vi "wait.vi"(1 "State to wait for":i32, 2 "Waiting Loop ID":i32, 3 "time (ms)":i32, 4 "Current Loop ID":i32) -> (0 "Done?":bool)   [LabVIEW 2013]
doc: "This VI allows you to wait for a specified amount of time before advancing, or for a different subsystem to reach a different state. Useful in autonomous applications."
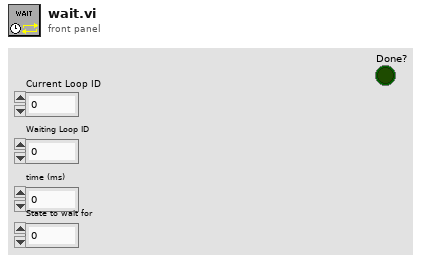
[diagram p1: front panel]
types:
  T1 = typedef "subStates.ctl" = enum16{"null", "wait", "driver control", "auto", "manual override", "hold position", "rotate", "pickup", "pass", "recover pass", "load", "goto shoot", "shoot high goal", "shoot low goal", "cancel arm", "cancel shooter", "end", "test"}
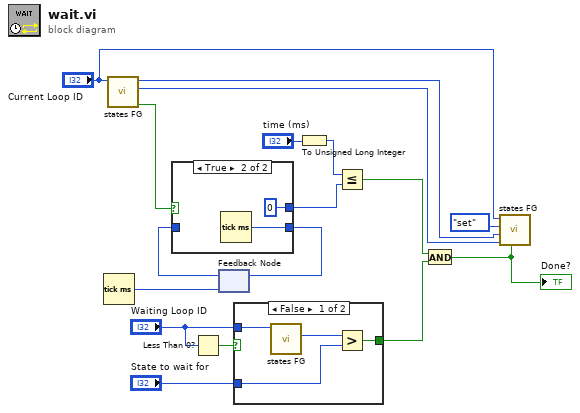
[diagram p0: block diagram]
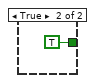
[diagram p2: hidden frame]
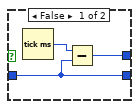
[diagram p3: hidden frame]
diagram:
  n1 = Tick Count (ms)() -> (millisecond timer value=w1:u32)
  n2 = call "states FG.vi"("Loop ID"="Current Loop ID") -> ("first call?"=w17:bool, "state # out"=w6:i32, "subState out"=w7:T1)  [unwired: 7 in, 1 out]
  n3 = Less Than 0?(x="Waiting Loop ID") -> (x < 0?=w2:bool)
  n4 = feedback #1(w1) -> (w15:u32)
  n5 = case shown="True" w17 {
    tunnel: [w19 w22] -> w16
    tunnel: w15 -> [w19 _]
    tunnel: [w18 u32 0] -> w14
    frame False {
      n6 = Tick Count (ms)() -> (millisecond timer value=w20:u32)
      n7 = Subtract(x=w20, y=w19) -> (x-y=w18:u32)
    }
    frame True {
      n8 = Tick Count (ms)() -> (millisecond timer value=w22:u32)
    }
  }
  n9 = feedback-in #1(w16) -> ()
  n10 = case shown="False" w2 {
    tunnel: "Waiting Loop ID" -> [w26 _]
    tunnel: "State to wait for" -> [w25 _]
    tunnel: [w24 TRUE] -> w11
    frame False {
      n11 = call "states FG.vi"("Loop ID"=w26) -> ("state # out"=w23:i32)  [unwired: 7 in, 3 out]
      n12 = Greater?(x=w23, y=w25) -> (0:w24:bool)
    }
    frame True {
    }
  }
  n13 = To Unsigned Long Integer(number="time (ms)") -> (unsigned 32bit integer=w4:u32)
  n14 = Less Or Equal?(x=w4, y=w14) -> (x <= y?=w12:bool)
  n15 = And(x=w12, y=w11) -> (x .and. y?=w10:bool)
  "Done?" <- w10
  n16 = call "states FG.vi"("exit in"=w10, "state # in"=w6, "subState in"=w7, "menu (get)"=enum16{"set", "get"}."set", "Loop ID"="Current Loop ID") -> ()  [unwired: 3 in, 4 out]
